vi "MirrorTrue.vi"(6 "Dest Format":string(combo)="{6fddc324-4e03-4bfe-b185-3d77768dc90e}", 7 "HTTP_address":string, 10 "Value":T3, 11 "Refnum in":T2) -> (3 "headers":string)   [LabVIEW 2016]
uses:
  cgi_string.ctl
  <vilib>/httpClient/ClientHandle.ctl
  <vilib>/vision/Image Controls.llb/IMAQ Image.ctl
  <vilib>/httpClient/LabVIEWHTTPClient.lvlib
panel:
  out "AuthorizationHeader":string
  in  "password":string="gamma2018"
  in  "Username":string="admin"
  out "Dest Format":string(combo)="{6fddc324-4e03-4bfe-b185-3d77768dc90e}"
  out "Image":T1(plugin-control)
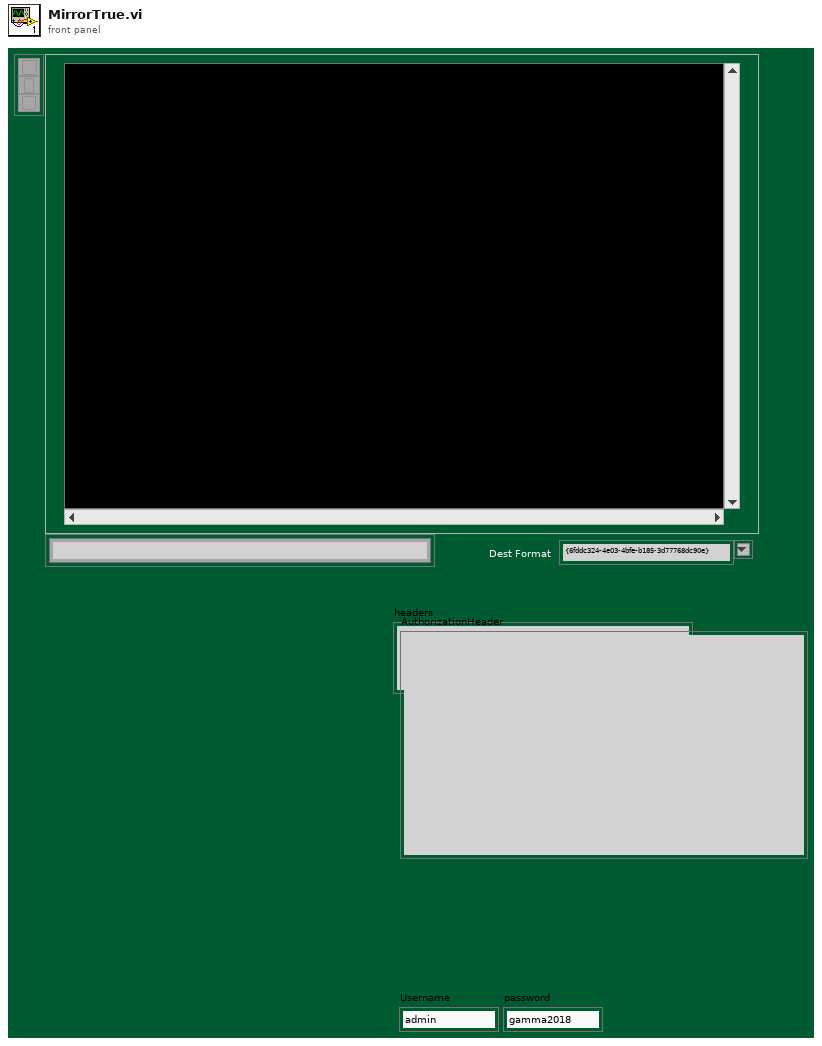
[diagram p1: front panel]
types:
  T1 = typedef "IMAQ Image.ctl" = refnum<image>
  T2 = typedef "LabVIEWHTTPClient.lvlib/ClientHandle.ctl" = refnum<k1>
  T3 = typedef "cgi_string.ctl" = string
  T4 = typedef "Image Type" = u32
  T5 = cluster{"realm":string, "qop":string, "nounce":string, "opaque":string}
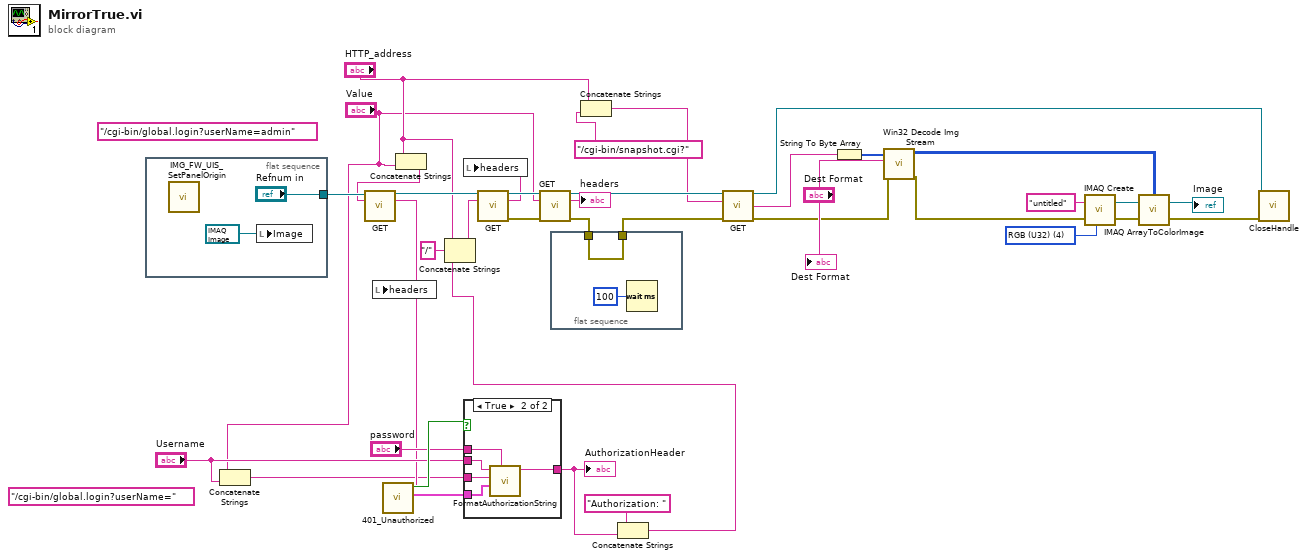
[diagram p0: block diagram]
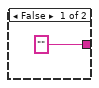
[diagram p2: hidden frame]
diagram:
  (unwired) "/cgi-bin/global.login?userName="
  (unwired) "/cgi-bin/global.login?userName=admin" ("string")
  w37 = T4 4 items=["Grayscale (U8)", "Grayscale (I16)", "Grayscale (SGL)", "Complex (CSG)", "RGB (U32)", "HSL (U32)", "RGB (U64)", "Grayscale (U16)"] ("Image Type")
  n1 = flat-sequence {
    tunnel: ["Refnum in"] -> w19
    frame #0 {
      n2 = call "IMG_FW_UIS_SetPanelOrigin.vi"() -> ()  [unwired: 11 in, 1 out]
      n3 = local write "Image"(T1 refnum ("New Image")) -> ()
    }
  }
  n4 = Concatenate Strings("Value", "Username") -> (w7:string)
  n5 = Concatenate Strings("HTTP_address", "Value") -> (w8:string)
  n6 = call <vilib>:"GET.vi"("client handle"=w19, "url"=w8) -> ("client handle out"=w17:T2, "headers"=w9:string)  [unwired: 10 in, 2 out]
  n7 = local write "headers"(w9) -> ()
  n8 = call "401_Unauthorized.vi"("headers"=w9) -> ("ServerInfo"=w14:T5, "401?"=w15:bool)  [unwired: 8 in, 1 out]
  n9 = case shown="True" w15 {
    tunnel: w14 -> [_ w46]
    tunnel: "Username" -> [_ w45]
    tunnel: w7 -> [_ w43]
    tunnel: "password" -> [_ w44]
    tunnel: ["" w42] -> w10
    frame False {
    }
    frame True {
      n10 = call "FormatAuthorizationString.vi"("password"=w44, "ServerInfo"=w46, "String in"=w43, "Username"=w45) -> ("String out"=w42:string)  [unwired: 7 in]
    }
  }
  "AuthorizationHeader" <- w10
  n11 = flat-sequence {
    tunnel: [w48] -> w21
    tunnel: w22 -> [w48]
    frame #0 {
      n12 = Wait (ms)(milliseconds to wait=u32 100) -> ()  [unwired: 1 out]
    }
  }
  n13 = Concatenate Strings("HTTP_address", "/cgi-bin/snapshot.cgi?") -> (w23:string)
  n14 = Concatenate Strings("Authorization: " ("string"), w10) -> (w6:string)
  n15 = Concatenate Strings("HTTP_address", "/" ("string"), w6) -> (w5:string)
  n16 = call <vilib>:"GET.vi"("client handle"=w17, "url"=w5) -> ("client handle out"=w16:T2, "headers"=w2:string, "error out"=w18:errorcluster)  [unwired: 10 in, 1 out]
  n17 = local write "headers"(w2) -> ()
  n18 = call <vilib>:"GET.vi"("client handle"=w16, "url"="Value", "error in (no error)"=w18) -> ("client handle out"=w27:T2, "headers"=→"headers":string, "error out"=w22:errorcluster)  [unwired: 9 in, 1 out]
  n19 = call <vilib>:"GET.vi"("client handle"=w27, "url"=w23, "error in (no error)"=w21) -> ("client handle out"=w26:T2, "body"=w28:string, "error out"=w25:errorcluster)  [unwired: 9 in, 1 out]
  n20 = String To Byte Array(string=w28) -> (unsigned byte array=w35:u8[])
  n21 = call "Win32 Decode Img Stream.vi"("error in (no error)"=w25, "Dest Format"="Dest Format", "Image Data"=w35) -> ("error out"=w32:errorcluster, "Dest"=w34:u32[][])  [unwired: 4 in, 3 out]
  n22 = call "IMAQ Create"("Image Name"="untitled", "Image Type"=w37, "error in (no error)"=w32) -> ("New Image"=w38:T1, "error out"=w33:errorcluster)  [unwired: 2 in]
  n23 = call "IMAQ ArrayToColorImage"("Image Pixels (U32)"=w34, "Image"=w38, "error in (no error)"=w33) -> ("Image Out"=→"Image":T1, "error out"=w29:errorcluster)  [unwired: 2 in]
  n24 = call <vilib>:"CloseHandle.vi"("client handle"=w26, "error in (no error)"=w29) -> ()  [unwired: 13 in, 1 out]
  "Dest Format" <- "Dest Format"
